vi "Test.vi"() -> ()   [LabVIEW 2024]
uses:
  System.Drawing
  C:/Users/Andrey/Desktop/wpf_bounds_test/WpfBoundsTestProps/Release/WindowsFormsControlLibrary.dll
  WindowsFormsControlLibrary.dll
panel:
  out "ToString 2":string
  in  "B":i32(slide) scale=0.0..255.0
  in  "G":i32(slide) scale=0.0..255.0
  in  "R":i32(slide) scale=0.0..255.0
  out "running":i32
  out "ToArgb":i32
  out "ToString":string
  in  "Stop Button":bool
  out "error out":errorcluster
  in  "UserControl1":refnum<k24>(container)
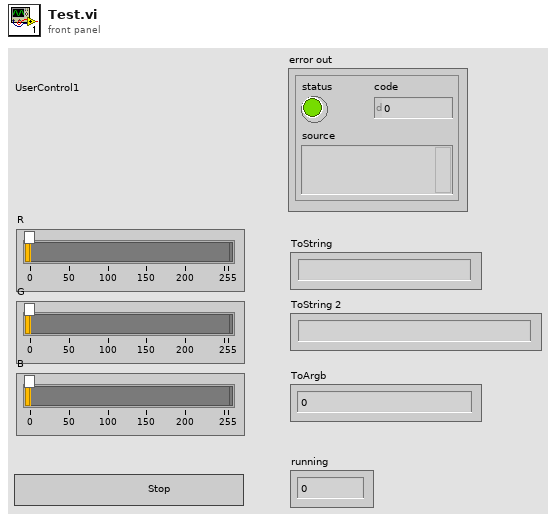
[diagram p1: front panel]
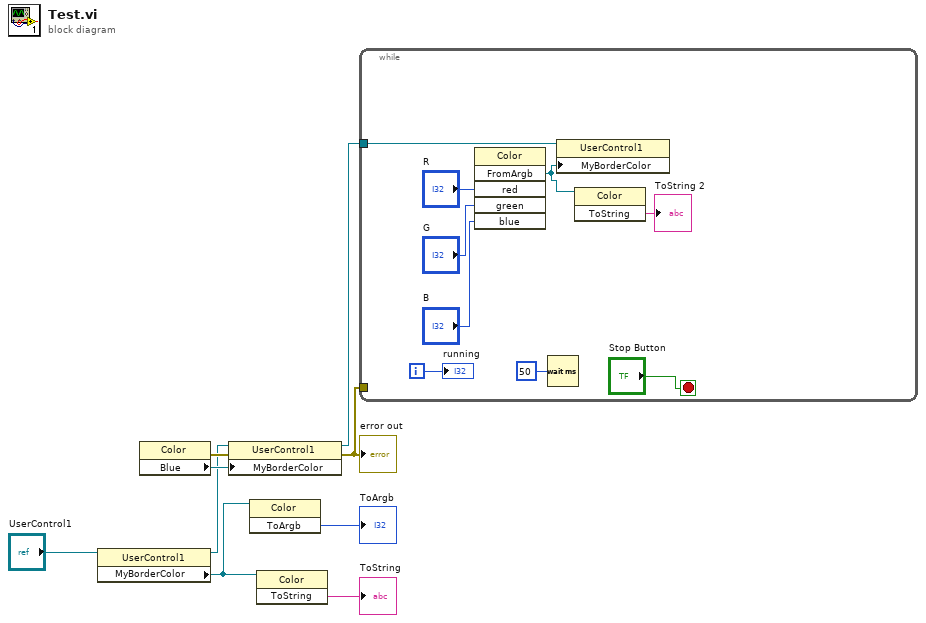
[diagram p0: block diagram]
diagram:
  n1 = property class="UserControl1"(reference="UserControl1") -> (reference out=w5:refnum<k24>, "MyBorderColor"=w3:refnum<k24>)  [unwired: 1 in, 1 out]
  n2 = property class="Color"() -> (error out=w8:errorcluster, "Blue"=w9:refnum<k24>)  [unwired: 2 in, 1 out]
  n3 = property class="UserControl1"(reference=w5, error in=w8, "MyBorderColor"=w9) -> (reference out=w1:refnum<k24>, error out=w7:errorcluster)
  "error out" <- w7
  n4 = invoke class="Color" method="ToArgb"(reference=w3) -> ("ToArgb"=→"ToArgb":i32)  [unwired: 2 in, 2 out]
  n5 = invoke class="Color" method="ToString"(reference=w3) -> ("ToString"=→"ToString":string)  [unwired: 2 in, 2 out]
  n6 = while {
    tunnel: w7 -> [_]
    tunnel: w1 -> [w16]
    i -> [w15]
    stop <- "Stop Button" stop-if-true
    n7 = invoke class="Color" method="FromArgb"("red"="R", "green"="G", "blue"="B") -> ("FromArgb"=w11:refnum<k24>)  [unwired: 3 in, 5 out]
    n8 = Wait (ms)(milliseconds to wait=u32 50) -> ()  [unwired: 1 out]
    n9 = property class="UserControl1"(reference=w16, "MyBorderColor"=w11) -> ()  [unwired: 1 in, 2 out]
    n10 = invoke class="Color" method="ToString"(reference=w11) -> ("ToString"=→"ToString 2":string)  [unwired: 2 in, 2 out]
    "running" <- w15
  }
